vi "ReversedEngineering CheckCtlStereoType.vi"(1 "TypeDefPath":path) -> (0 "ClassDesc":string)   [LabVIEW 2016]
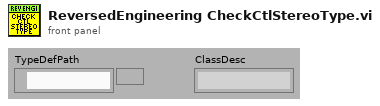
[diagram p1: front panel]
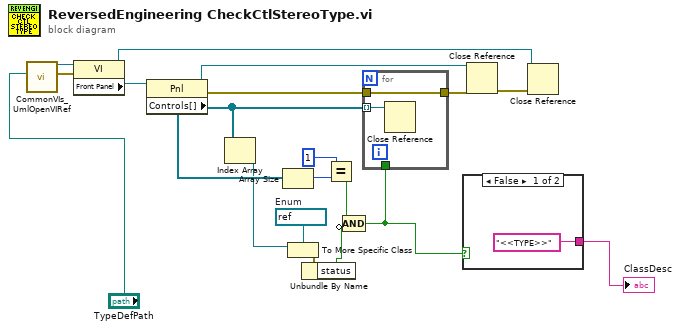
[diagram p0: block diagram]
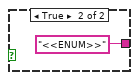
[diagram p2: hidden frame]
diagram:
  w6 = refnum<vi> refnum  # Enum
  n1 = call <resource>:"CommonVIs_UmlOpenVIRef.vi"("ViPath/ViName"="TypeDefPath") -> ("error out"=w3:errorcluster, "vi reference"=w2:refnum<vi>)  [unwired: 3 in, 6 out]
  n2 = property class="VI"(reference=w2, error in=w3) -> (reference out=w19:refnum<vi>, "Front Panel"=w5:refnum<vi>)  [unwired: 1 out]
  n3 = property class="Pnl"(reference=w5) -> (reference out=w17:refnum<vi>, error out=w16:errorcluster, "Controls[]"=w13:refnum<vi>[])  [unwired: 1 in]
  n4 = Index Array(array=w13) -> (element=w12:refnum<vi>)  [unwired: 1 in]
  n5 = Array Size(array=w13) -> (size(s)=w8:i32)
  n6 = To More Specific Class(target class=w6, reference=w12) -> (error out=w7:errorcluster)  [unwired: 1 in, 1 out]
  n7 = Unbundle By Name(w7) -> ("status"=w10:bool)
  n8 = Equal?(x=1, y=w8) -> (x = y?=w11:bool)
  n9 = Compound Arithmetic op=AND(w11, invert w10) -> (w14:bool)
  n10 = for {
    tunnel: w13 -> [w21] mode=indexing
    tunnel: w14 -> [_]
    tunnel: [w20] -> w15
    tunnel: w16 -> [w20]
    n11 = Close Reference(reference=w21) -> ()  [unwired: 1 in, 1 out]
  }
  n12 = case shown="False" w14 {
    tunnel: ["<<TYPE>>" ("ClassDesc") "<<ENUM>>" ("ClassDesc")] -> w4
    frame False {
    }
    frame True {
    }
  }
  "ClassDesc" <- w4
  n13 = Close Reference(reference=w17, error in (no error)=w15) -> (error out=w18:errorcluster)
  n14 = Close Reference(reference=w19, error in (no error)=w18) -> ()  [unwired: 1 out]
